vi "HEWH Config Read.vi"(0 "Config File Path":path=path "C:/work/flowconfig.ini", 11 "error in (no error)":errorcluster) -> (6 "found?":bool, 15 "error out":errorcluster)   [LabVIEW 2012]
uses:
  HEWH Error Enumeration.ctl
  <vilib>/Utility/config.llb/Read Key (String).vi
  Global HEWH.vi
  <vilib>/Utility/config.llb/NI_LVConfig.lvlib
panel:
  out "Array":bool[](array[boolean])
  out "Tank Flow (GPM,Percent)":dbl[][](array[numeric])
  out "Purge Flow (GPM,Percent)":dbl[][](array[numeric])
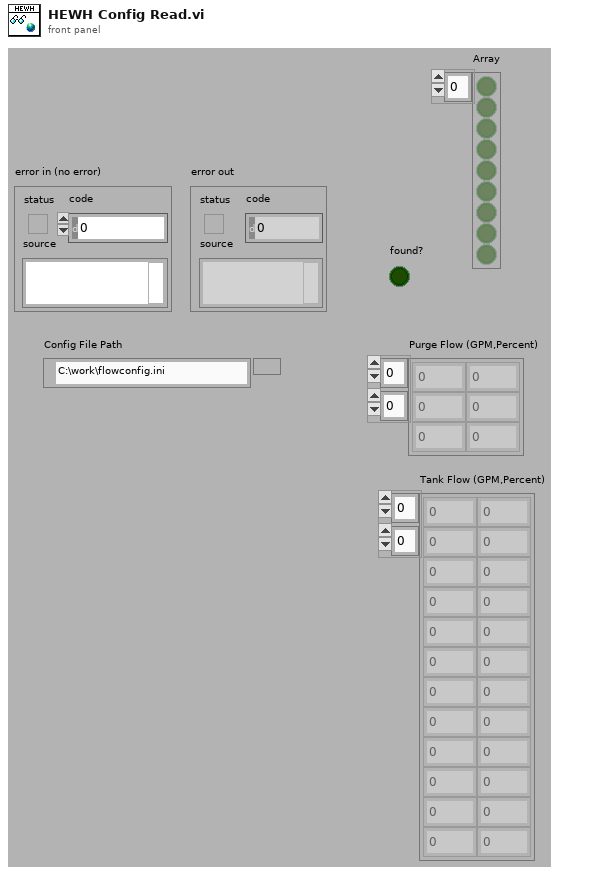
[diagram p1: front panel]
types:
  T1 = typedef "NI_LVConfig.lvlib/Config Data RefNum.ctl" = refnum<k1>
  T2 = typedef "HEWH Error Enumeration.ctl" = enum16{"No Error", "GEA2 Send ACK Mismatch", "GEA2 STX", "GEA2 ETX", "GEA2 CRC Mismatch", "GEA2 ReadACK", "RTD In Range Error", "Fail Mean Tank Temp", "No Flow Config Data Found", "Failed Flow During Purge", "Temp During Purge", "Confirm IF Stop Fail", "Init Draw: TC_1 Out of Range", "Flow = 0 During Draw after 20s"}
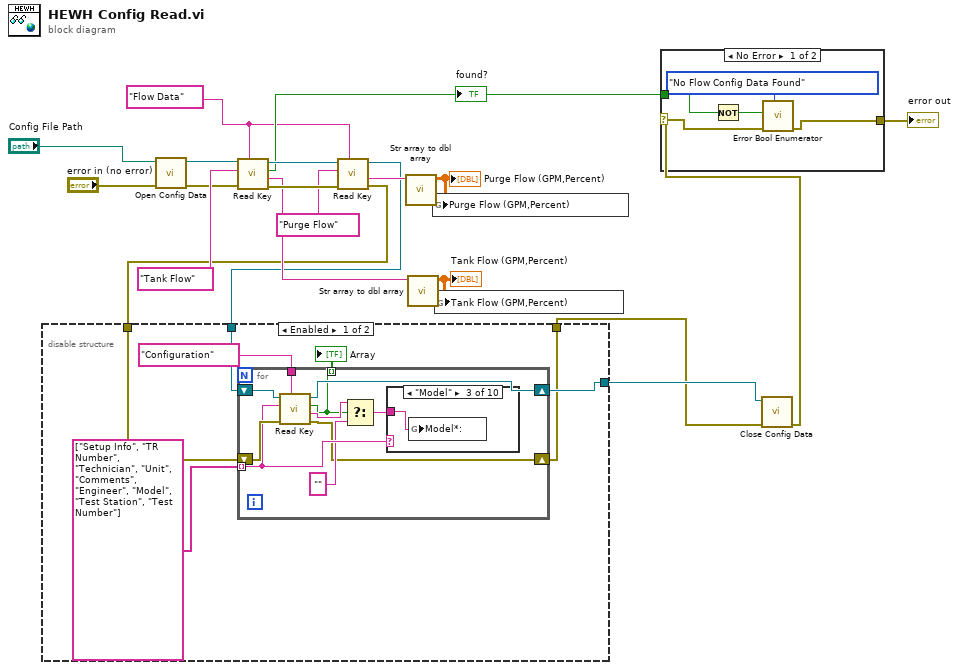
[diagram p0: block diagram]
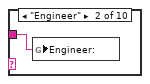
[diagram p3: hidden frame]
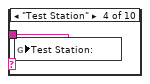
[diagram p4: hidden frame]
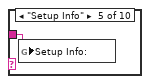
[diagram p5: hidden frame]
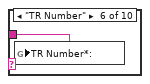
[diagram p6: hidden frame]
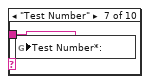
[diagram p7: hidden frame]
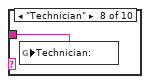
[diagram p8: hidden frame]
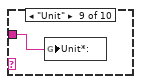
[diagram p9: hidden frame]
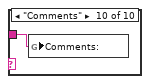
[diagram p10: hidden frame]
diagram:
  w9 = "Flow Data" ("section")
  n1 = call <vilib>:"Open Config Data.vi"("error in (no error)"="error in (no error)", "configuration file path"="Config File Path") -> ("error out"=w4:errorcluster, "refnum"=w19:T1)  [unwired: 7 in, 1 out]
  n2 = call-poly <vilib>:"Read Key.vi"("section"=w9, "error in (no error)"=w4, "key"="Tank Flow", "refnum"=w19) -> ("error out"=w20:errorcluster, "value"=w15:string, "found?"=w10:bool, "refnum out"=w18:T1)  [unwired: 4 in]
  "found?" <- w10
  n3 = call-poly <vilib>:"Read Key.vi"("section"=w9, "error in (no error)"=w20, "key"="Purge Flow", "refnum"=w18) -> ("error out"=w3:errorcluster, "value"=w14:string, "refnum out"=w5:T1)  [unwired: 4 in, 1 out]
  n4 = disable-structure shown="Enabled" {
    disable-tunnel: w3 -> [w25 _]
    disable-tunnel: [w24 _] -> w6
    disable-tunnel: w5 -> [w23 _]
    disable-tunnel: [w22 _] -> w2
    frame Enabled {
      n5 = for {
        tunnel: "Configuration" ("key") -> [w35]
        tunnel: string[] ["Setup Info", "TR Number", "Technician", "Unit", "Comments", "Engineer", "Model", "Test Station", "Test Number"] -> [w34] mode=indexing
        shift-right: [w29] -> w22
        shift-left: w25 -> [w36]
        shift-right: [w30] -> w24
        shift-left: w23 -> [w37]
        tunnel: [w28] -> w21 mode=indexing
        n6 = call-poly <vilib>:"Read Key.vi"("section"=w35, "error in (no error)"=w36, "key"=w34, "refnum"=w37) -> ("error out"=w29:errorcluster, "value"=w33:string, "found?"=w28:bool, "refnum out"=w30:T1)  [unwired: 4 in]
        n7 = Select(t=w33, s=w28, f="") -> (s? t:f=w32:string)
        n8 = case shown="\"Model\"" w34 {
          tunnel: w32 -> [_ w38 w39 w40 w41 w42 w43 w44 w45 w46]
          frame "False", Default {
          }
          frame "Engineer" {
            n9 = global write "Global HEWH.vi" "Engineer:"(w38) -> ()
          }
          frame "Model" {
            n10 = global write "Global HEWH.vi" "Model*:"(w39) -> ()
          }
          frame "Test Station" {
            n11 = global write "Global HEWH.vi" "Test Station:"(w40) -> ()
          }
          frame "Setup Info" {
            n12 = global write "Global HEWH.vi" "Setup Info:"(w41) -> ()
          }
          frame "TR Number" {
            n13 = global write "Global HEWH.vi" "TR Number*:"(w42) -> ()
          }
          frame "Test Number" {
            n14 = global write "Global HEWH.vi" "Test Number*:"(w43) -> ()
          }
          frame "Technician" {
            n15 = global write "Global HEWH.vi" "Technician:"(w44) -> ()
          }
          frame "Unit" {
            n16 = global write "Global HEWH.vi" "Unit*:"(w45) -> ()
          }
          frame "Comments" {
            n17 = global write "Global HEWH.vi" "Comments:"(w46) -> ()
          }
        }
      }
      "Array" <- w21
    }
    frame Disabled {
    }
  }
  n18 = call "Str array to dbl array.vi"("String array in"=w14) -> ("Double array out"=w13:dbl[][])  [unwired: 9 in, 1 out]
  "Purge Flow (GPM,Percent)" <- w13
  n19 = call "Str array to dbl array.vi"("String array in"=w15) -> ("Double array out"=w12:dbl[][])  [unwired: 9 in, 1 out]
  "Tank Flow (GPM,Percent)" <- w12
  n20 = global write "Global HEWH.vi" "Purge Flow (GPM,Percent)"(w13) -> ()
  n21 = global write "Global HEWH.vi" "Tank Flow (GPM,Percent)"(w12) -> ()
  n22 = call <vilib>:"Close Config Data.vi"("error in (no error)"=w2, "refnum"=w6) -> ("error out"=w1:errorcluster)  [unwired: 8 in, 1 out]
  n23 = case shown="No Error" w1 {
    selector: w1 -> [w50 w52]
    tunnel: [w51 w52] -> w11
    tunnel: w10 -> [w48 _]
    frame No Error {
      n24 = Not(x=w48) -> (.not. x?=w47:bool)
      n25 = call "Error Bool Enumerator.vi"("Error Enum"=HEWH_Error_Enumeration."No Flow Config Data Found", "Error In"=w50, "Error?"=w47) -> ("Error Out"=w51:errorcluster)  [unwired: 6 in]
    }
    frame Error {
    }
  }
  "error out" <- w11
